vi "ZZZ un horror Chroma 1905x Series Measure Statistics POP.vi"(5 "error in":T1, 8 "inst handle in":refnum<visa-resource-name>) -> (0 "error out":T1, 1 "Current":string, 2 "Status":string caption="Result", 3 "inst handle out":refnum<visa-resource-name>, 4 "Complete Test":string)   [LabVIEW 2025]
doc: "Contact Chroma\nTEL: +886-2-2298-3855 \nTEL: +886-3-397-5788 \nFAX: +886-2-2298-3596\nFAX: +886-3-327-4703 \nURL: http://www.chromaate.com \nE-mail: chroma@chroma.com.tw"
panel:
  out "Check Equipment":bool
  out "?":dbl(graph)
  out "Current/Resistance":string
  out "Actual Voltage":string
  out "Test Voltage":string
  out "Current value":dbl format="%.2f"
  out "array4":dbl[](array[numeric]) format="%.5f"
  out "Lo Current Limit":string
  out "Hi Current Limit":string
  out "Fail":dbl
  out "Pass copy":dbl
  out "Abort":dbl
  out "Sum":dbl
  out "current limit string":string
  out "array1":i32[](array[numeric]) format="%.5f"
  out "array3":dbl[](array[numeric]) format="%.5f"
  out "array2":dbl[](array[numeric]) format="%.5f"
  out "Counter":dbl format="%.2f"
  out "Voltage":string
  out "Testing":bool
  out "Failure":bool
  out "Pass":bool
  out "Testing/Danger":bool
  out "refnum copy 2":refnum<file>
  in  "FINISHED":bool
  in  "MEASURE":bool
  out "refnum copy":refnum<file>
  out "Step":string
  # "This is designed for measurements on the Chroma 1905x with single step"
  # "DANGER"
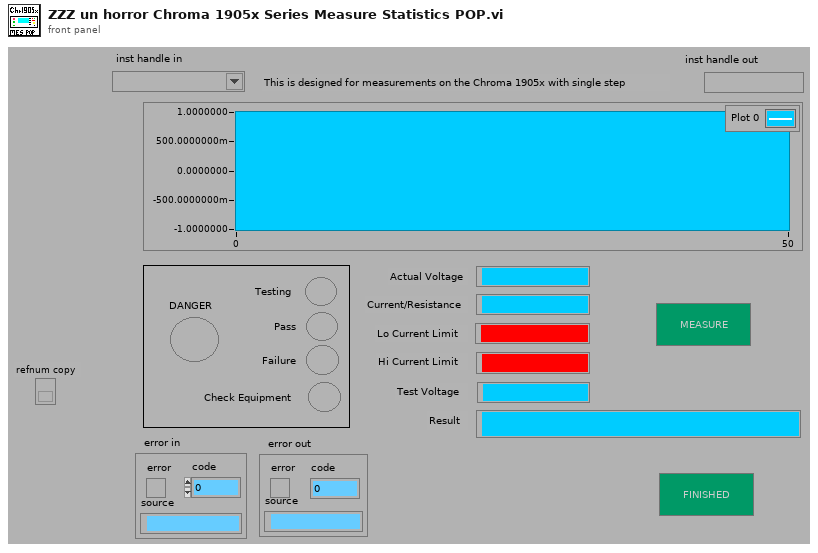
[diagram p1: front panel]
types:
  T1 = cluster{"error":bool, "code":i8, "source":string}
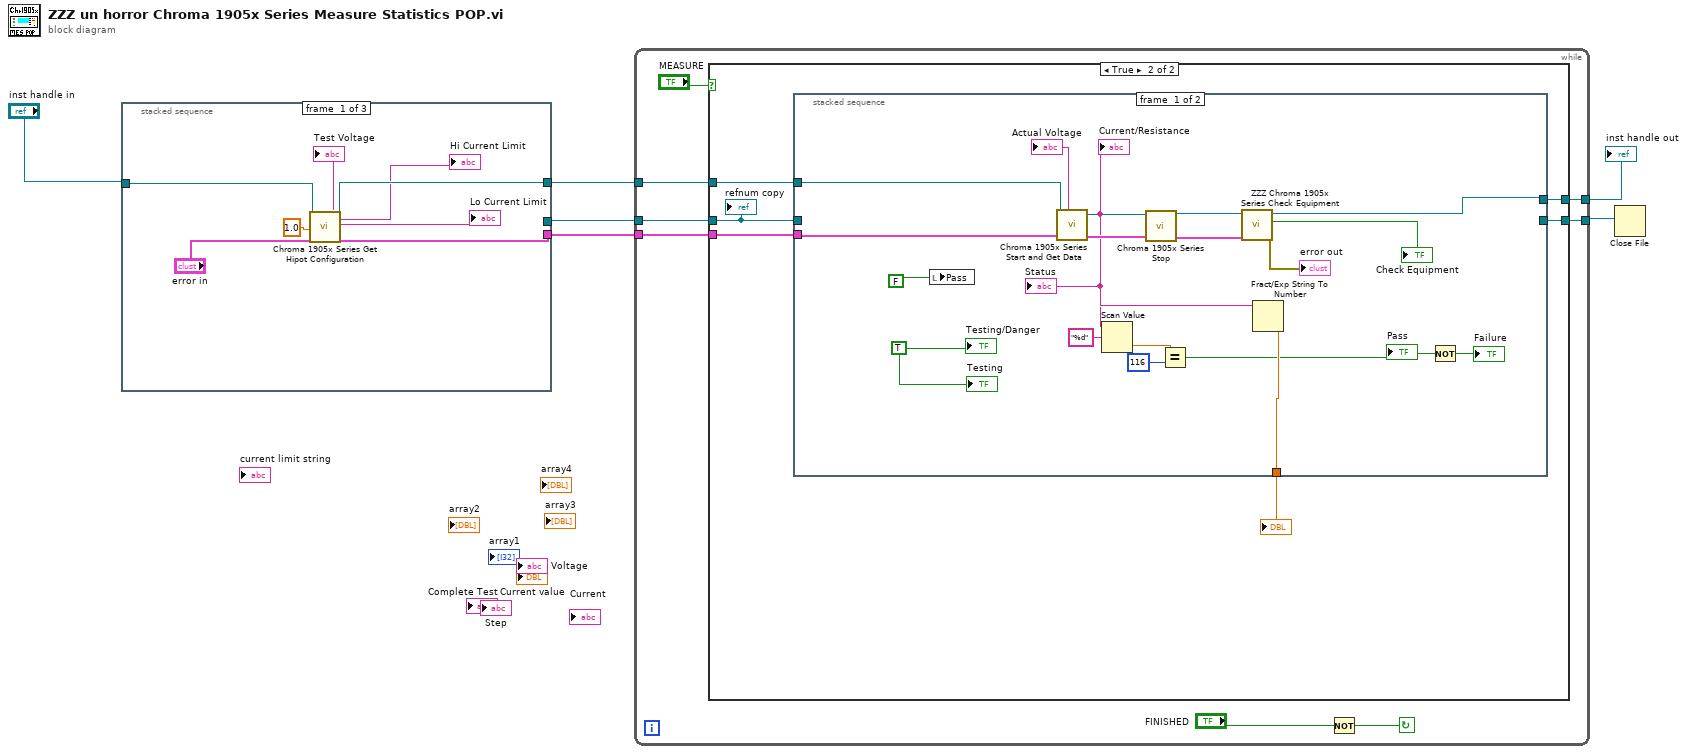
[diagram p0: block diagram]
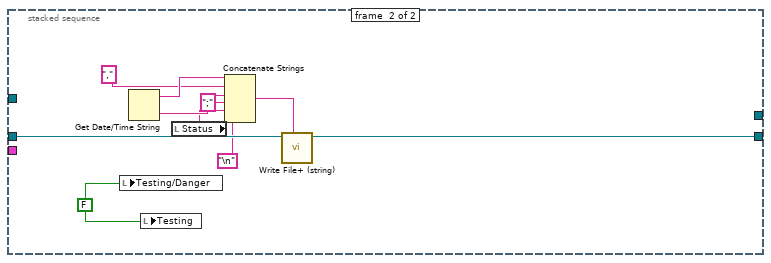
[diagram p3: hidden frame]
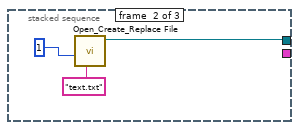
[diagram p4: hidden frame]
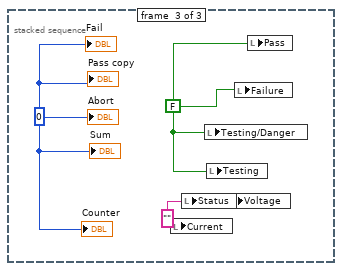
[diagram p5: hidden frame]
diagram:
  n1 = stacked-sequence {
    tunnel: [_ w15 _] -> w5
    tunnel: [w12 _ _] -> w4
    tunnel: "inst handle in" -> [w13 _ _]
    tunnel: [w10 _ _] -> w3
    frame #0 {
      n2 = call "Chroma 1905x Series Get Hipot Configuration.vi"("inst handle in"=w13, "Step Number"=1.0, "error in"="error in") -> ("Voltage Level"=→"Test Voltage":string, "inst handle out"=w12:refnum<visa-resource-name>, "Hi Limit"=→"Hi Current Limit":string, "Low Limit"=→"Lo Current Limit":string, "error out"=w10:T1)  [unwired: 5 in, 7 out]
    }
    frame #1 {
      n3 = call <vilib>:"Open_Create_Replace File.vi"("default name"="text.txt", "function (open:0)"=i16 1 ("open or create file")) -> ("refnum"=w15:refnum<file>)  [unwired: 6 in, 3 out]
    }
    frame #2 {
      w18 = ""
      w19 = FALSE
      w20 = 0
      n4 = local write "Current"(w18) -> ()
      n5 = local write "Status"(w18) -> ()
      n6 = local write "Testing/Danger"(w19) -> ()
      n7 = local write "Testing"(w19) -> ()
      n8 = local write "Voltage"(w18) -> ()
      n9 = local write "Failure"(w19) -> ()
      n10 = local write "Pass"(w19) -> ()
      "Sum" <- w20
      "Abort" <- w20
      "Pass copy" <- w20
      "Fail" <- w20
      "Counter" <- w20
    }
  }
  n11 = while {
    tunnel: [w21] -> w2
    tunnel: w3 -> [w22]
    tunnel: w4 -> [w23]
    tunnel: [w24] -> w6
    tunnel: w5 -> [w27]
    stop <- w25 continue-if-true
    n12 = case shown="True" "MEASURE" {
      tunnel: w27 -> [w30 w36]
      tunnel: [w30 w35] -> w24
      tunnel: w23 -> [w29 w34]
      tunnel: w22 -> [_ w33]
      tunnel: [w29 w31] -> w21
      frame False {
      }
      frame True {
        n13 = stacked-sequence {
          tunnel: w36 -> [_ w65]
          tunnel: [_ w65] -> w35
          tunnel: w34 -> [w48 _]
          tunnel: w33 -> [w47 _]
          tunnel: [w56 _] -> w32
          tunnel: [w51 _] -> w31
          frame #0 {
            w55 = TRUE
            n14 = local write "Pass"(FALSE) -> ()
            n15 = call "Chroma 1905x Series Start and Get Data.vi"("inst handle in"=w48, "error in"=w47) -> ("Voltage"=→"Actual Voltage":string, "Current"=w44:string, "inst handle out"=w45:refnum<visa-resource-name>, "Judgement Last Test"=w42:string, "error out"=w46:T1)  [unwired: 2 in, 1 out]
            "Status" <- w42
            "Current/Resistance" <- w44
            n16 = Scan Value(string=w42, format string="%d") -> (value=w40:dbl)  [unwired: 1 in, 1 out]
            n17 = call "Chroma 1905x Series Stop.vi"("error in"=w46, "inst handle in"=w45) -> ("error out"=w53:T1, "inst handle out"=w52:refnum<visa-resource-name>)  [unwired: 1 in]
            n18 = Equal?(x=w40, y=i16 116) -> (x = y?=w38:bool)
            "Pass" <- w38
            n19 = call "ZZZ Chroma 1905x Series Check Equipment.vi"("error in (no error)"=w53, "inst handle in"=w52) -> ("error out"=→"error out":errorcluster, "Equipment Error"=→"Check Equipment":bool, "inst handle out"=w51:refnum<visa-resource-name>)  [unwired: 7 in]
            n20 = Fract/Exp String To Number(string=w44) -> (number=w56:dbl)  [unwired: 3 in, 1 out]
            n21 = Not(x=w38) -> (.not. x?=→"Failure":bool)
            "Testing/Danger" <- w55
            "Testing" <- w55
          }
          frame #1 {
            w61 = FALSE
            n22 = local write "Testing/Danger"(w61) -> ()
            n23 = Get Date/Time String() -> (date string=w64:string, time string=w63:string)  [unwired: 3 in]
            n24 = local write "Testing"(w61) -> ()
            n25 = local read "Status"() -> (w59:string)
            n26 = Concatenate Strings(w64, ",", w63, ";" ("Substring"), w59, "\n") -> (w62:string)
            n27 = call <vilib>:"Write File+ (string).vi"("string"=w62, "refnum"=w65) -> ()  [unwired: 5 in, 3 out]
          }
        }
        "?" <- w32
        "refnum copy" <- w36
      }
    }
    n28 = Not(x="FINISHED") -> (.not. x?=w25:bool)
  }
  "inst handle out" <- w2
  n29 = Close File(refnum=w6) -> ()  [unwired: 1 in, 2 out]
